vi "GetAllParam.vi"(7 "group":string, 8 "error in (no error)":errorcluster, 11 "_ConfigClass_INI_IN":refnum<class "_ConfigClass_INI.lvclass">) -> (0 "error out":errorcluster, 2 "params":string[](array[string]), 3 "_ConfigClass_INI_OUT":refnum<class "_ConfigClass_INI.lvclass">)   [LabVIEW 2019, in "_ConfigClass_INI.lvlib" / "_ConfigClass_INI.lvclass"]
uses:
  _ConfigClass_INI.lvclass
  <vilib>/Utility/config.llb/NI_LVConfig.lvlib
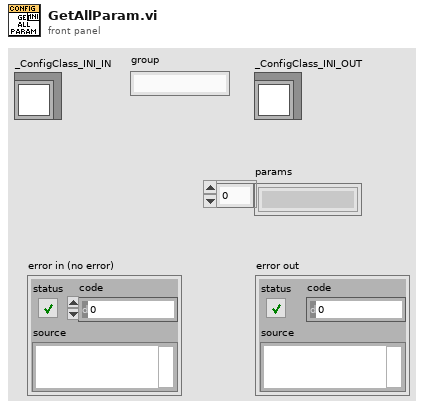
[diagram p1: front panel]
types:
  T1 = typedef "NI_LVConfig.lvlib/Config Data RefNum.ctl" = refnum<k1>
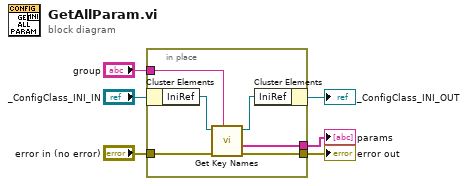
[diagram p0: block diagram]
diagram:
  n1 = in-place {
    in-place-border: "group" -> [w11]
    in-place-border: [w9] -> w4
    in-place-border: [w8] -> w3
    in-place-border: "error in (no error)" -> [w7]
    n2 = in-place-cluster #1("_ConfigClass_INI_IN") -> ("IniRef"=w12:T1)
    n3 = call <vilib>:"Get Key Names.vi"("section"=w11, "error in (no error)"=w7, "refnum"=w12) -> ("error out"=w8:errorcluster, "key names"=w9:string[], "refnum out"=w10:T1)  [unwired: 5 in, 1 out]
    n4 = in-place-cluster #1("IniRef"=w10) -> (→"_ConfigClass_INI_OUT":refnum<class "_ConfigClass_INI.lvclass">)
  }
  "error out" <- w3
  "params" <- w4
